vi "ROS2 Read.vi"(10 "DDS in":u64[](array[numeric]), 11 "error in":errorcluster[](array[cluster])) -> (1 "error out":errorcluster[](array[cluster]), 2 "Amplified Read":dbl[](array[numeric]), 3 "DDS out":u64[](array[numeric]))   [LabVIEW 2021]
uses:
  <vilib>/RTI DDS Toolkit/VIs/Read_NumI32.vi
  <vilib>/RTI DDS Toolkit/Library/LVDDS_library.lvlib
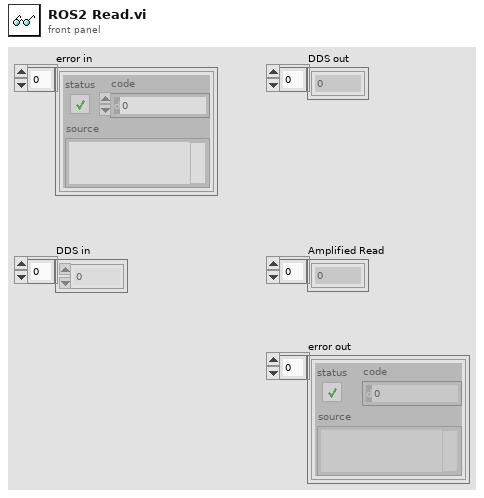
[diagram p1: front panel]
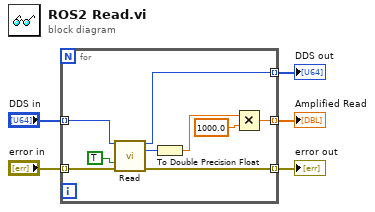
[diagram p0: block diagram]
diagram:
  n1 = for {
    tunnel: [w10] -> w3 mode=indexing
    tunnel: [w9] -> w4 mode=indexing
    tunnel: [w8] -> w5 mode=indexing
    tunnel: "DDS in" -> [w7] mode=indexing
    tunnel: "error in" -> [w6] mode=indexing
    n2 = call-poly <vilib>:"Read.vi"("DDS Object Ref in"=w7, "Only New Samples"=TRUE, "error in (no error)"=w6) -> ("DDS Object Ref out"=w9:u64, "Data"=w14:i32, "error out"=w10:errorcluster)  [unwired: 8 in, 2 out]
    n3 = To Double Precision Float(number=w14) -> (double precision float=w13:dbl)
    n4 = Multiply(x=w13, y=1000.0) -> (x*y=w8:dbl)
  }
  "Amplified Read" <- w5
  "DDS out" <- w4
  "error out" <- w3
